vi "Configure Serial Bus (CXPI - Basic).vi"(0 "VISA resource name":refnum<visa-resource-name>, 1 "Tolerance (4%)":i32=4, 5 "Serial Bus Name (1: Serial Bus 1)":i32(ring)=1 items=["Serial Bus 1"=1, "Serial Bus 2"=2], 7 "Source Channel (0: Channel 1)":i32(ring) items=["Channel 1", "Channel 2", "Channel 3", "Channel 4"], 9 "Baud Rate (20000 bps)":i32=20000, 11 "error in (no error)":errorcluster, 12 "Enable Parity Bits (F: Disable)":bool) -> (4 "VISA resource name out":refnum<visa-resource-name>, 15 "error out":errorcluster)   [LabVIEW 2017, in "Agilent 2000 3000 X-Series.lvlib"]
doc: "Configures the basic setting of CXPI bus.\n\n<b>Note:</b>\nThis VI is only applicable for 3000T, 4000, 6000 X-Series."
uses:
  Agilent 2000 3000 X-Series.lvlib
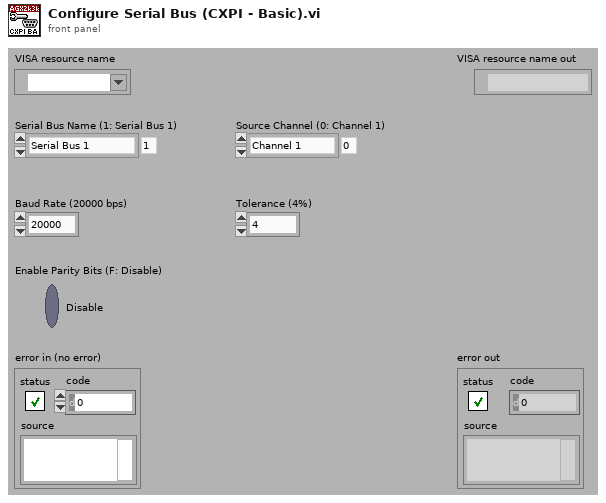
[diagram p1: front panel]
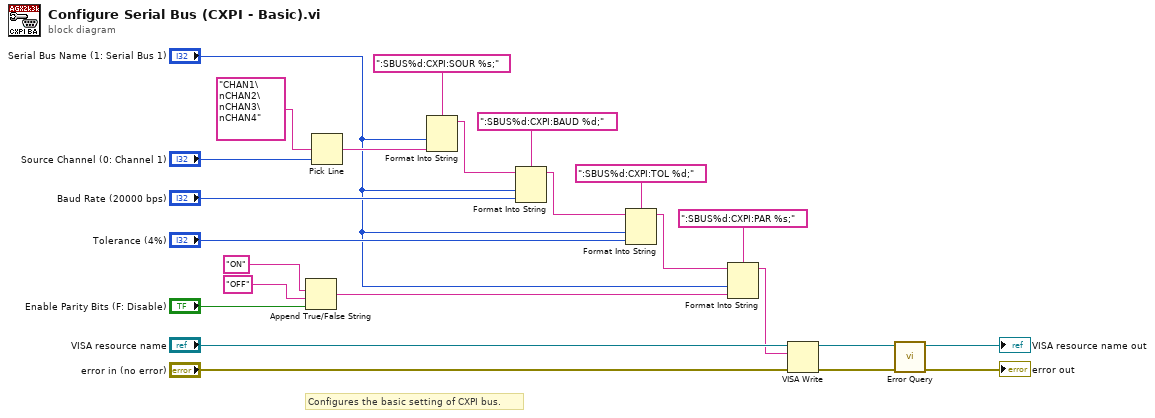
[diagram p0: block diagram]
diagram:
  # "Configures the basic setting of CXPI bus."
  n1 = Append True/False String(1:"Enable Parity Bits (F: Disable)", 2:"OFF", 3:"ON") -> (0:w20:string)  [unwired: 1 in]
  n2 = Pick Line(multi-line string="CHAN1\nCHAN2\nCHAN3\nCHAN4", line index="Source Channel (0: Channel 1)") -> (output string=w18:string)  [unwired: 1 in]
  n3 = Format Into String(format string=":SBUS%d:CXPI:SOUR %s;", "Serial Bus Name (1: Serial Bus 1)", w18) -> (resulting string=w9:string)  [unwired: 2 in, 1 out]
  n4 = Format Into String(format string=":SBUS%d:CXPI:BAUD %d;", initial string=w9, "Serial Bus Name (1: Serial Bus 1)", "Baud Rate (20000 bps)") -> (resulting string=w8:string)  [unwired: 1 in, 1 out]
  n5 = Format Into String(format string=":SBUS%d:CXPI:TOL %d;", initial string=w8, "Serial Bus Name (1: Serial Bus 1)", "Tolerance (4%)") -> (resulting string=w6:string)  [unwired: 1 in, 1 out]
  n6 = Format Into String(format string=":SBUS%d:CXPI:PAR %s;", initial string=w6, "Serial Bus Name (1: Serial Bus 1)", w20) -> (resulting string=w5:string)  [unwired: 1 in, 1 out]
  n7 = VISA Write(VISA resource name="VISA resource name", write buffer=w5, error in (no error)="error in (no error)") -> (VISA resource name out=w4:refnum<visa-resource-name>, error out=w3:errorcluster)  [unwired: 1 out]
  n8 = call "Error Query.vi"("error in (no error)"=w3, "VISA resource name"=w4) -> ("error out"=→"error out":errorcluster, "VISA resource name out"=→"VISA resource name out":refnum<visa-resource-name>)  [unwired: 6 in, 2 out]
